vi "GetImageType.vi"(8 "error in (no error)":errorcluster, 11 "CameraTesting in":refnum<class "CameraTesting.lvclass">) -> (0 "error out":errorcluster, 3 "CameraTesting out":refnum<class "CameraTesting.lvclass">)   [LabVIEW 2020, in "CameraTesting.lvlib" / "CameraTesting.lvclass"]
uses:
  CameraTesting.lvclass
  CameraTesting.lvclass/CameraTesting.ctl
  Camera/ICamera/ICamera/ICamera.lvclass
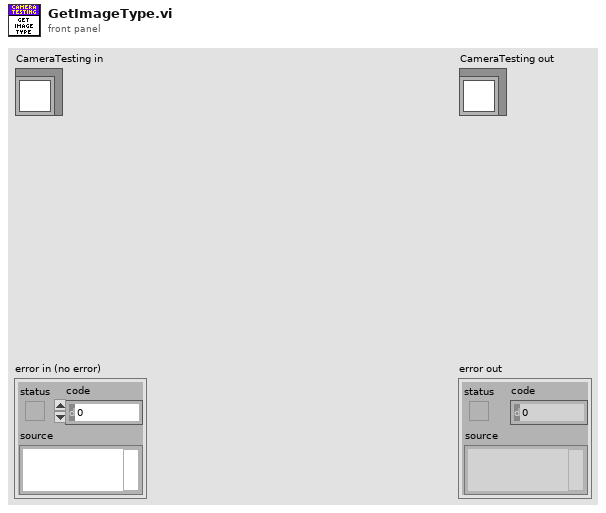
[diagram p1: front panel]
types:
  T1 = typedef "ICameraTesting.lvlib/ICameraTesting.lvclass/ImgTypeValReceived.ctl" = refnum<user-event>
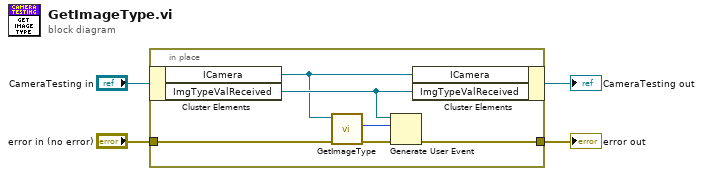
[diagram p0: block diagram]
diagram:
  n1 = in-place {
    in-place-border: "error in (no error)" -> [w6]
    in-place-border: [w9] -> w3
    n2 = in-place-cluster #1("CameraTesting in") -> ("ICamera"=w8:refnum<class "ICamera.lvclass">, "ImgTypeValReceived"=w10:T1)
    n3 = call-dynamic "GetImageType.vi"("error in (no error)"=w6, "ICamera in"=w8) -> ("error out"=w5:errorcluster, "Image Type"=w7:u8)  [unwired: 7 in, 1 out]
    n4 = Generate User Event(user event=w10, event data cluster=w7, error in=w5) -> (error out=w9:errorcluster)  [unwired: 1 in, 1 out]
    n5 = in-place-cluster #1("ICamera"=w8, "ImgTypeValReceived"=w10) -> (→"CameraTesting out":refnum<class "CameraTesting.lvclass">)
  }
  "error out" <- w3
